vi "Action.vi"(8 "error in (no error)":errorcluster, 10 "Action":string, 11 "HarnessInterface in":refnum<class "_Class.lvclass">) -> (0 "error out":errorcluster, 3 "HarnessInterface out":refnum<class "_Class.lvclass">)   [LabVIEW 2021, in "_Class.lvlib" / "_Class.lvclass"]
uses:
  _Class.lvclass
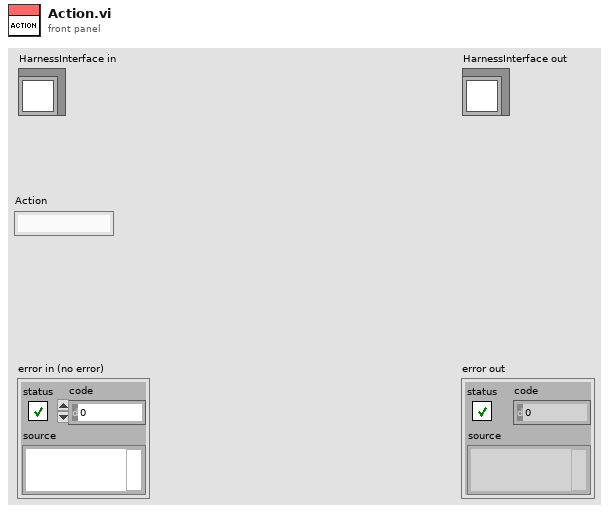
[diagram p1: front panel]
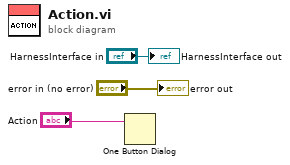
[diagram p0: block diagram]
diagram:
  n1 = One Button Dialog(message="Action") -> ()  [unwired: 1 in, 1 out]
  "error out" <- "error in (no error)"
  "HarnessInterface out" <- "HarnessInterface in"
